vi "About VI.vi"(10 "Model Name":string) -> ()   [LabVIEW 2014]
panel:
  out "About VI":string
  in  "Close":bool
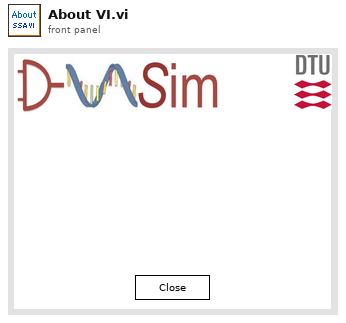
[diagram p1: front panel]
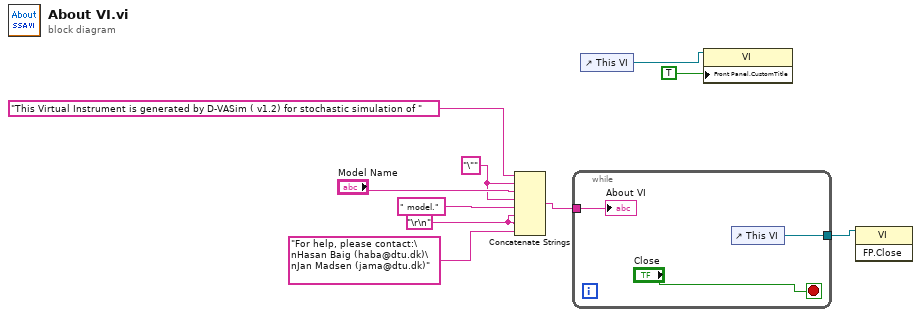
[diagram p0: block diagram]
diagram:
  w3 = "\r\n"
  w5 = "\"" ("string")
  n1 = Concatenate Strings("This Virtual Instrument is generated by D-VASim ( v1.2) for stochastic simulation of ", w5, "Model Name", w5, " model." ("string"), w3, w3, "For help, please contact:\nHasan Baig (haba@dtu.dk)\nJan Madsen (jama@dtu.dk)" ("string")) -> (w1:string)
  n2 = while {
    tunnel: [w12] -> w10
    tunnel: w1 -> [w11]
    stop <- "Close" stop-if-true
    n3 = control-ref of="This VI"() -> (w12:refnum<vi>)
    "About VI" <- w11
  }
  n4 = control-ref of="This VI"() -> (w9:refnum<vi>)
  n5 = property class="VI"(reference=w9, "Front Panel.CustomTitle"=TRUE ("Front Panel Window:Custom Title")) -> ()  [unwired: 1 in, 2 out]
  n6 = invoke class="VI" method="FP.Close"(reference=w10) -> ()  [unwired: 2 in, 3 out]
